vi "FormulaNodeExampleMarcoGonzalez.vi"() -> ()   [LabVIEW 2012]
panel:
  in  "stop":bool
  out "Z":dbl
  in  "Y":dbl
  in  "X":dbl
  # "Marco Gonzalez\nEA 3 / 02/02/2017\nFormular Node Example"
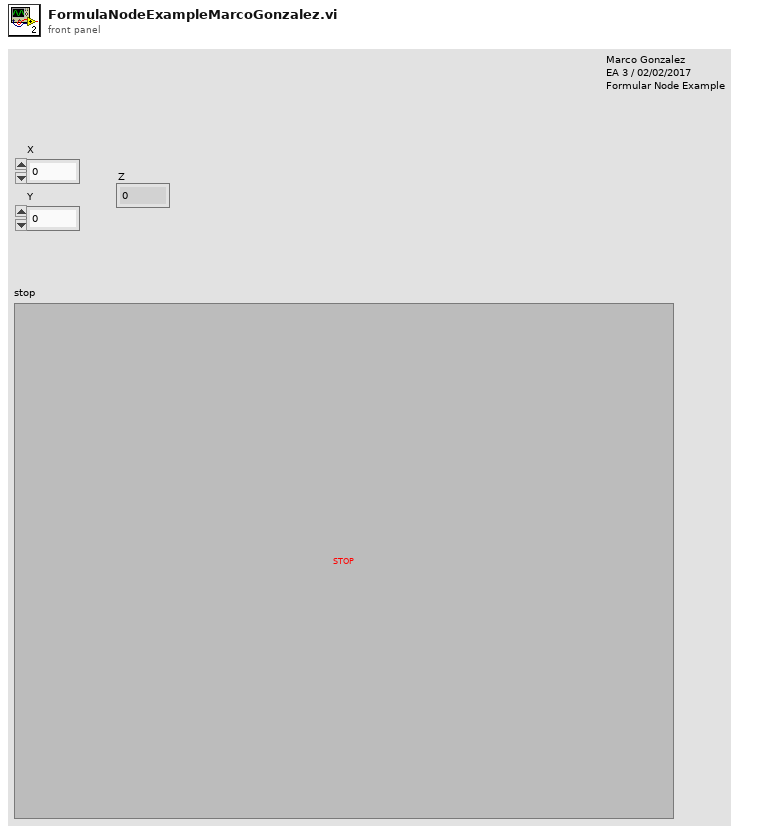
[diagram p1: front panel]
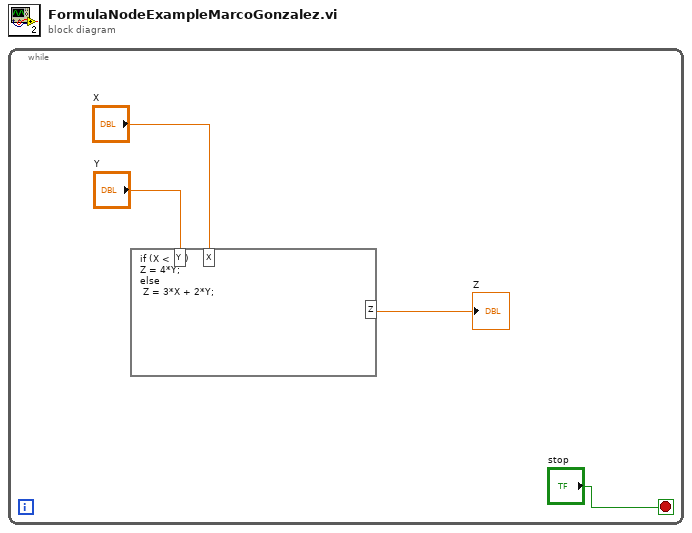
[diagram p0: block diagram]
diagram:
  n1 = while {
    stop <- "stop" stop-if-true
    n2 = formula code="if (X < 10)\nZ = 4*Y;\nelse\n Z = 3*X + 2*Y;"("X"="X", "Y"="Y") -> ("Z"=→"Z":dbl)
  }
